vi "TestXYGraph_MultiplotSinglePlot.vi"() -> ()   [LabVIEW 2019]
panel:
  out "XY Graph 2":cluster{dbl[], dbl[]}[](graph)
  out "CCD 1D Spectrum Main 2":cluster{dbl[], dbl[]}[](graph) caption="Main spectrum"
  out "XY Graph":cluster{dbl[], dbl[]}[](graph)
  in  "Y":dbl[](array[numeric])=[50.0, 40.0, 20.0, 80.0, 20.0, 20.0, 50.0, 30.0, 10.0, 40.0, 90.0, 40.0, 150.0, 200.0, 740.0, 1700.0, 1350.0, 880.0, 1120.0, 4110.0, 7840.0, 7780.0, 5250.0, 5060.0, 4520.0, 7060.0, 12990.0, 11660.0, 6970.0, 7230.0, 9730.0, 9730.0, 8500.0, 8990.0, 12820.0, 15270.0, 14910.0, 8050.0, 7540.0, 11050.0, 14810.0, 10180.0, 8220.0, 780.0, 900.0, 330.0, 210.0, 210.0, 190.0, 160.0, 150.0, 90.0, 60.0, 50.0, 70.0, 70.0, 90.0, 80.0, 70.0, 30.0, 40.0]
  in  "X":dbl[](array[numeric])=[2.7675044642857145, 2.767195625488227, 2.7668868556125865, 2.766578154635725, 2.766269522534583, 2.765960959286113, 2.7656524648672764, 2.7653440392550466, 2.7650356824264053, 2.7647273943583457, 2.764419175027871, 2.7641110244119944, 2.7638029424877395, 2.763494929232141, 2.763186984622242, 2.7628791086350977, 2.762571301247772, 2.7622635624373397, 2.761955892180887, 2.7616482904555077, 2.7613407572383077, 2.7610332925064025, 2.7607258962369183, 2.7604185684069913, 2.7601113089937668, 2.759804117974402, 2.759496995326063, 2.7591899410259266, 2.7588829550511798, 2.758576037379019, 2.758269187986652, 2.757962406851296, 2.757655693950178, 2.757349049260536, 2.757042472759618, 2.7567359644246805, 2.756429524232993, 2.7561231521618317, 2.755816848188487, 2.7555106122902546, 2.755204444444445, 2.7548983446283746, 2.7545923128193737, 2.7542863489947798, 2.7539804531319416, 2.753674625208218, 2.753368865200977, 2.7530631730875985, 2.752757548845471, 2.752451992451993, 2.752146503884573, 2.7518410831206306, 2.7515357301375944, 2.751230444912904, 2.7509252274240072, 2.7506200776483642, 2.7503149955634427, 2.750009981146723, 2.7497050343756935, 2.7494001552278524, 2.7490953436807097]
  in  "CCD 1D Spectrum Main":cluster{dbl[], dbl[]}(graph)={array[1340 elements], array[1340 elements]} caption="Main spectrum"
  # "211221\n\nTest pour essayer de comprendre comment passer de A à B selon les données à plot\n\n\nA = plot XY i.e. un bundle de X et Y\n\nB = 2 plots XY i.e. un array de bundles de X et Y"
  # "Conclusion:\n\nTout dépend du dernier \"truc\" qui a été passé au terminal du XYGraph (pas les variables locales mais bien le terminal)\n\nEt passer A (ou B) puis B (ou A) ne donne plus d'erreur lorsque c'est fait directement sur le terminal"
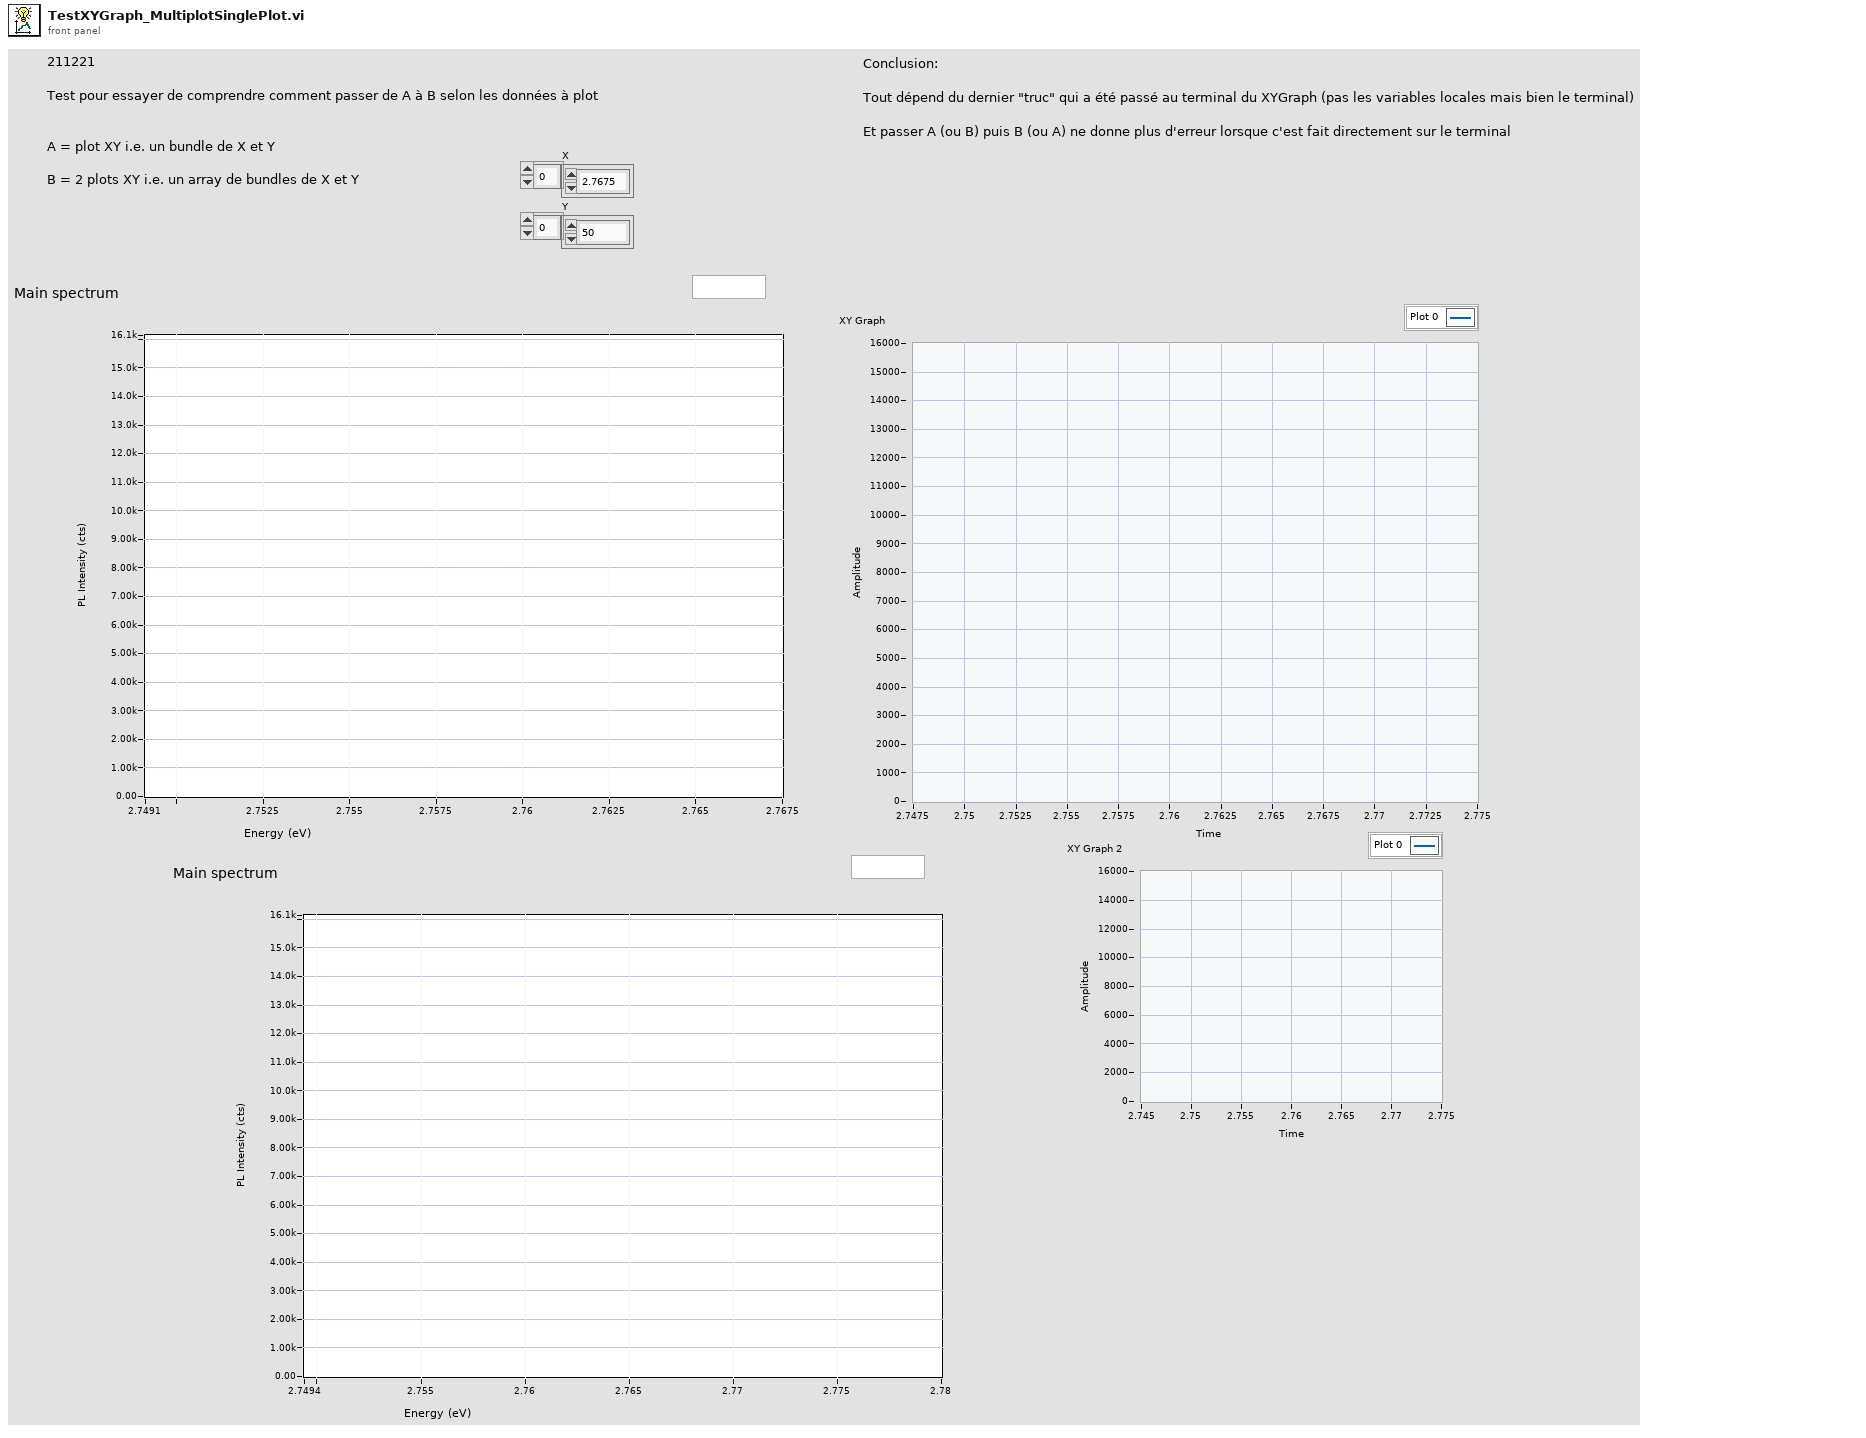
[diagram p1: front panel]
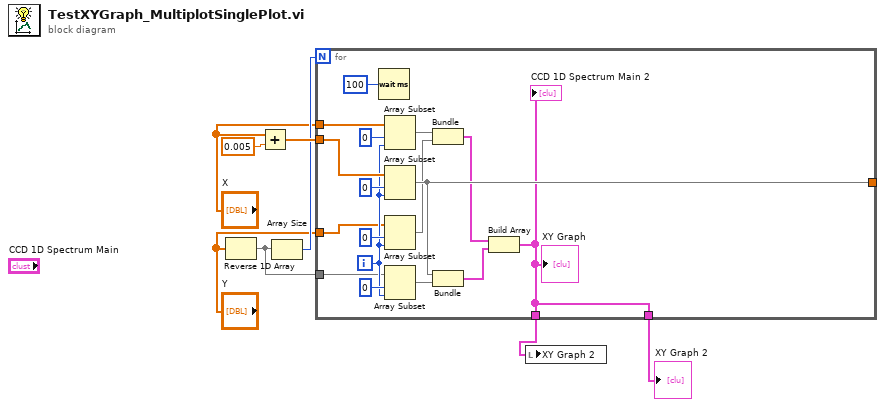
[diagram p0: block diagram]
diagram:
  n1 = Reverse 1D Array(array="Y") -> (reversed array=w6:dbl[])
  n2 = Add(x="X", y=0.005) -> (x+y=w7:dbl[])
  n3 = Array Size(array=w6) -> (size(s)=w5:i32)
  n4 = for {
    N: w5 -> [_]
    tunnel: w6 -> [w12]
    tunnel: w7 -> [w25]
    tunnel: [w22] -> _
    tunnel: "X" -> [w18]
    tunnel: "Y" -> [w13]
    tunnel: [w9] -> w2
    tunnel: [w9] -> w1
    i -> [w16]
    n5 = Wait (ms)(milliseconds to wait=u32 100) -> ()  [unwired: 1 out]
    n6 = Array Subset(array=w18, index=0, length=w16) -> (w14:dbl[])
    n7 = Array Subset(array=w25, index=0, length=w16) -> (w22:dbl[])
    n8 = Array Subset(array=w13, index=0, length=w16) -> (w15:dbl[])
    n9 = Array Subset(array=w12, index=0, length=w16) -> (w21:dbl[])
    n10 = Bundle(w14, w15) -> (w10:cluster{dbl[], dbl[]})  [unwired: 1 in]
    n11 = Bundle(w22, w21) -> (w11:cluster{dbl[], dbl[]})  [unwired: 1 in]
    n12 = Build Array(w10, w11) -> (w9:cluster{dbl[], dbl[]}[])
    "XY Graph" <- w9
    "CCD 1D Spectrum Main 2" <- w9
  }
  "XY Graph 2" <- w1
  n13 = local write "XY Graph 2"(w2) -> ()
